vi "CreateString.vi"(11 "length":i32) -> (3 "string":string)   [LabVIEW 2025, in "LibZMQ.lvlib"]
doc: "Create string of fixed length"
uses:
  LibZMQ.lvlib
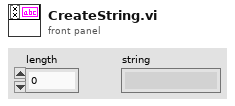
[diagram p1: front panel]
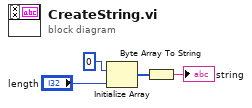
[diagram p0: block diagram]
diagram:
  n1 = Initialize Array(u8 0, "length") -> (w2:u8[])
  n2 = Byte Array To String(unsigned byte array=w2) -> (string=→"string":string)
